vi "Get Alarm State.vi"(0 "reference in":refnum<class "PM_Group.lvclass">) -> (4 "alarm state":bool)   [LabVIEW 2019, in "PM_Group.lvclass"]
uses:
  PM_Group.lvclass
  PM_Group.lvclass/PM_Group.ctl
  Engine_1DO_2DI_class/Engine_1DO_2DI.lvclass/Engine_1DO_2DI.ctl
  Sig_DA_class/Sig_DA.lvclass/Sig_DA.ctl
  Engine_1DO_2DI_class/Engine_1DO_2DI.lvclass
  Sig_DA_class/Sig_DA.lvclass
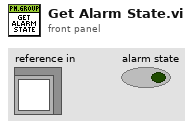
[diagram p1: front panel]
types:
  T1 = typedef "bool_data.ctl" = cluster{"CURR":bool, "RAW_PREV":bool, "millisecond timer value":u32}
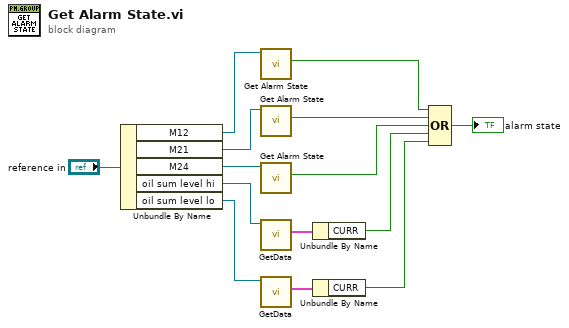
[diagram p0: block diagram]
diagram:
  n1 = Unbundle By Name("reference in") -> ("M12"=w8:refnum<class "Engine_1DO_2DI.lvclass">, "M21"=w9:refnum<class "Engine_1DO_2DI.lvclass">, "M24"=w10:refnum<class "Engine_1DO_2DI.lvclass">, "oil sum level hi"=w5:refnum<class "Sig_DA.lvclass">, "oil sum level lo"=w3:refnum<class "Sig_DA.lvclass">)
  n2 = call "Get Alarm State.vi"("Pump_1AI_1DO_2DI in"=w8) -> ("Alarm State"=w11:bool)  [unwired: 10 in]
  n3 = call "Get Alarm State.vi"("Pump_1AI_1DO_2DI in"=w9) -> ("Alarm State"=w12:bool)  [unwired: 10 in]
  n4 = call "Get Alarm State.vi"("Pump_1AI_1DO_2DI in"=w10) -> ("Alarm State"=w13:bool)  [unwired: 10 in]
  n5 = call "GetData.vi"("Sig_DA in"=w5) -> ("data"=w6:T1)  [unwired: 10 in]
  n6 = call "GetData.vi"("Sig_DA in"=w3) -> ("data"=w4:T1)  [unwired: 10 in]
  n7 = Unbundle By Name(w6) -> ("CURR"=w1:bool)
  n8 = Unbundle By Name(w4) -> ("CURR"=w2:bool)
  n9 = Compound Arithmetic op=OR(w11, w12, w13, w1, w2) -> (→"alarm state":bool)
